vi "NI VeriStand - Set Custom Device Drivers.vi"(6 "Version":string, 7 "Execution mode":T5, 8 "error in (no error)":errorcluster, 9 "Driver VI":T1[](array[typedef]), 11 "Device Ref in":T6 format="%.0x") -> (0 "error out":errorcluster, 3 "Device Ref out":T6 format="%.0x")   [LabVIEW 2020, in "Custom Device Offline API.lvlib"]
uses:
  <vilib>/NI VeriStand/Custom Device Offline API/Custom Device Offline API.lvlib
  <vilib>/NI VeriStand/Custom Device API/Custom Device Item Ref.ctl
  <vilib>/NI VeriStand/Custom Device API/Custom Device Execution Mode.ctl
  <vilib>/NI VeriStand/Custom Device API/Custom Device Path Data.ctl
  <vilib>/NI VeriStand/Custom Device API/Custom Device Supported Target.ctl
  <vilib>/NI VeriStand/Custom Device API/Path Specification.ctl
  <vilib>/NI VeriStand/Custom Device API/Path Type.ctl
  NationalInstruments.VeriStand.SystemDefinitionAPI
  <vilib>/NI VeriStand/Custom Device API/Custom Device API.lvlib
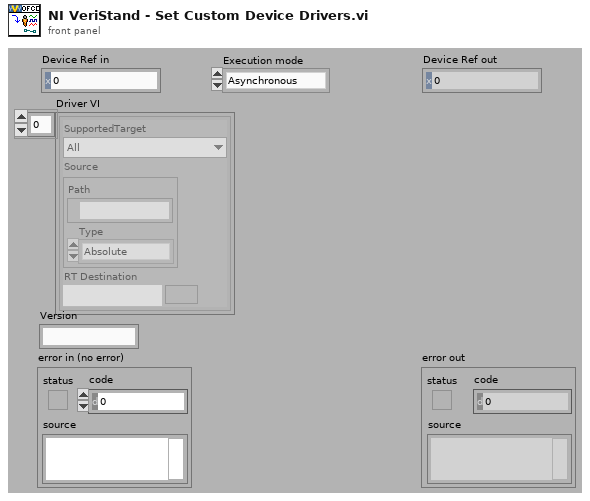
[diagram p1: front panel]
types:
  T1 = typedef "Custom Device API.lvlib/Custom Device Path Data.ctl" = cluster{"SupportedTarget":T2, "Source":T3, "RT Destination":path}
  T2 = typedef "Custom Device API.lvlib/Custom Device Supported Target.ctl" = enum16{"All", "PharLap", "VxWorks", "Windows", "Linux_32_ARM", "Linux_x64", "PharLap & Windows", "PharLap & VxWorks", "VxWorks & Windows"}
  T3 = typedef "Custom Device API.lvlib/Path Specification.ctl" = cluster{"Path":path, "Type":T4}
  T4 = typedef "Custom Device API.lvlib/Path Type.ctl" = enum16{"Absolute", "To Base", "To Common Data Dir", "To Application Data Dir"}
  T5 = typedef "Custom Device API.lvlib/Custom Device Execution Mode.ctl" = enum16{"Asynchronous", "Inline HW Interface", "Inline Model Interface", "Inline Timing and Sync", "Asynchronous Timing and Sync"}
  T6 = typedef "Custom Device API.lvlib/Custom Device Item Ref.ctl" = u64
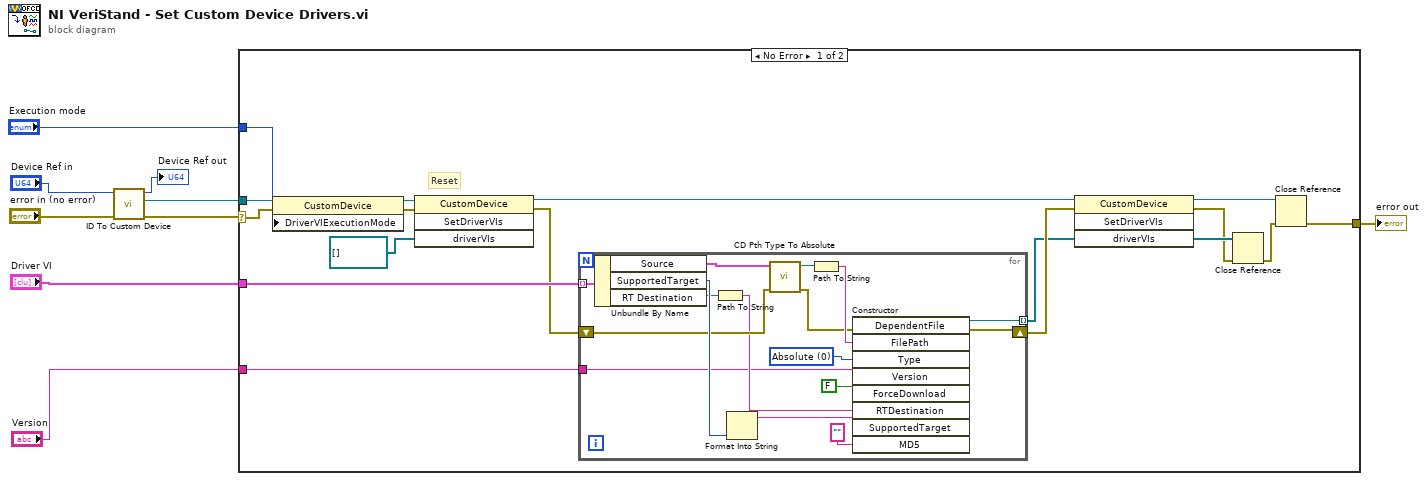
[diagram p0: block diagram]
diagram:
  n1 = call <vilib>:"ID To Custom Device.vi"("error in (no error)"="error in (no error)", "ID in"="Device Ref in") -> ("error out"=w6:errorcluster, "Device"=w5:refnum<k24>, "ID out"=→"Device Ref out":u64)  [unwired: 7 in]
  n2 = case shown="No Error" w6 {
    selector: w6 -> [w25 w43]
    tunnel: w5 -> [w26 _]
    tunnel: "Execution mode" -> [w24 _]
    tunnel: "Driver VI" -> [w23 _]
    tunnel: [w11 w43] -> w2
    tunnel: "Version" -> [w10 _]
    frame No Error {
      # "Reset"
      n3 = property class="CustomDevice"(reference=w26, error in=w25, "DriverVIExecutionMode"=w24) -> (reference out=w22:refnum<k24>, error out=w21:errorcluster)
      n4 = invoke class="CustomDevice" method="SetDriverVIs"(reference=w22, error in=w21, "driverVIs"=refnum<k24>[] []) -> (reference out=w18:refnum<k24>, error out=w19:errorcluster)  [unwired: 1 in, 2 out]
      n5 = for {
        tunnel: w23 -> [w42] mode=indexing
        shift-right: [w30] -> w17
        shift-left: w19 -> [w39]
        tunnel: [w29] -> w16 mode=indexing
        tunnel: w10 -> [w27]
        w34 = 0 items=["Absolute", "Relative", "ToCommonDocDir", "ToAppDataDir"] ("Type")
        n6 = Unbundle By Name(w42) -> ("Source"=w40:T3, "SupportedTarget"=w41:T2, "RT Destination"=w37:path)
        n7 = Path To String(path=w37) -> (string=w36:string)
        n8 = Format Into String(w41) -> (resulting string=w38:string)  [unwired: 3 in, 1 out]
        n9 = call <vilib>:"CD Pth Type To Absolute.vi"("error in (no error)"=w39, "CD Path Pair"=w40) -> ("error out"=w31:errorcluster, "Absolute Path"=w33:path)  [unwired: 8 in]
        n10 = Path To String(path=w33) -> (string=w32:string)
        n11 = constructor class="DependentFile"(error in=w31, "FilePath"=w32, "Type"=w34, "Version"=w27, "ForceDownload"=FALSE, "RTDestination"=w36, "SupportedTarget"=w38, "MD5"="" ("Version")) -> (reference out=w29:refnum<k24>, error out=w30:errorcluster)  [unwired: 2 in, 8 out]
      }
      n12 = invoke class="CustomDevice" method="SetDriverVIs"(reference=w18, error in=w17, "driverVIs"=w16) -> (reference out=w12:refnum<k24>, error out=w14:errorcluster, "driverVIs"=w15:refnum<k24>[])  [unwired: 1 in, 1 out]
      n13 = Close Reference(reference=w15, error in (no error)=w14) -> (error out=w13:errorcluster)
      n14 = Close Reference(reference=w12, error in (no error)=w13) -> (error out=w11:errorcluster)
    }
    frame Error {
    }
  }
  "error out" <- w2
